vi "Dm To Dkm.vi"(8 "error in (no error)":errorcluster, 11 "dMetres":dbl) -> (0 "error out":errorcluster, 3 "dkm":dbl)   [LabVIEW 2023, in "POSCONV.lvlib"]
doc: "Converts double metres to double kilometres (1km = 1000m)...\n\n\n\n\ndouble DmToDkm(double dMetres);"
uses:
  POSCONV.lvlib
  C:/Users/J Gordon/Documents/Rail Tech/TV-HR/02 - Code/Modules/POSCONV/POSCONV.dll
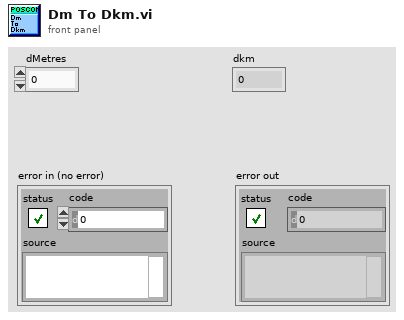
[diagram p1: front panel]
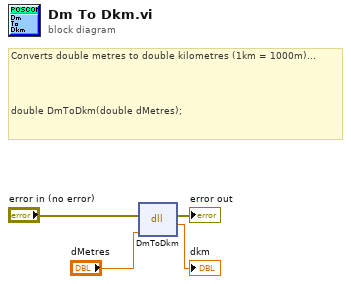
[diagram p0: block diagram]
diagram:
  # "Converts double metres to double kilometres (1km = 1000m)...\n\n\n\n\ndouble DmToDkm(double dMetres);"
  n1 = dll-call lib="C:/Users/J Gordon/Documents/Rail Tech/TV-HR/02 - Code/Modules/POSCONV/POSCONV.*" fn="DmToDkm"(error in="error in (no error)", "dMetres"="dMetres") -> (error out=→"error out":errorcluster, →"dkm":dbl)  [unwired: 3 in, 1 out]
